vi "Read Old.vi"(5 "channel list":string="BL_SELs", 6 "current limit range (A)":dbl=3.2e-05 format="%#_6p", 7 "aperture time (s)":dbl=0.0005 format="%#_6p", 8 "error in (no error)":errorcluster, 9 "settling time (s)":dbl=0.001 format="%#_6p", 10 "voltage level (V)":dbl=0.2 format="%#_6p", 11 "instrument handle":refnum<k15>="PXI1Slot2 (8)") -> (0 "error out":errorcluster, 1 "currents (A)":dbl[](array[numeric])=[9.855399817894821e-07, -1.469813883694186e-08, -9.562873863260234e-08, -9.678400506461213e-09, -4.0653341648640705e-08, -1.6774881378946392e-08, 2.609795137832926e-09, -3.578297908247983e-08], 2 "resistances (ohm)":dbl[](array[numeric])=[101467.21781741035, -6803582.488189799, -1045710.7500308217, -10332285.787640315, -2459822.3896151385, -5961294.016988207, 38317183.80893152, -2794624.7787111253], 3 "instrument handle out":refnum<k15>="PXI1Slot2 (8)")   [LabVIEW 2018]
uses:
  <instrlib>/niDigital/niDigital.llb/niDigital Selected Function.ctl
  Globals.vi
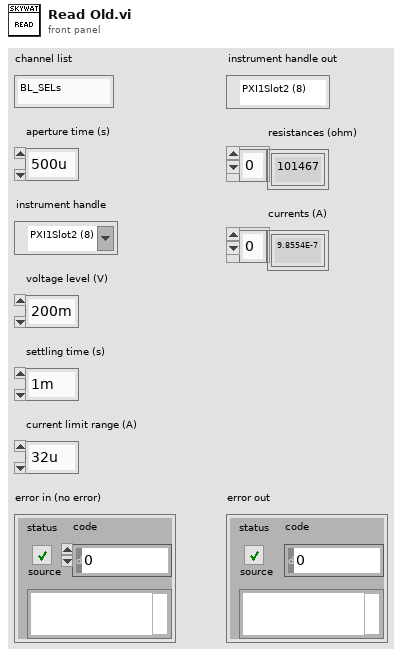
[diagram p1: front panel]
types:
  T1 = typedef "niDigital Selected Function.ctl" = i32
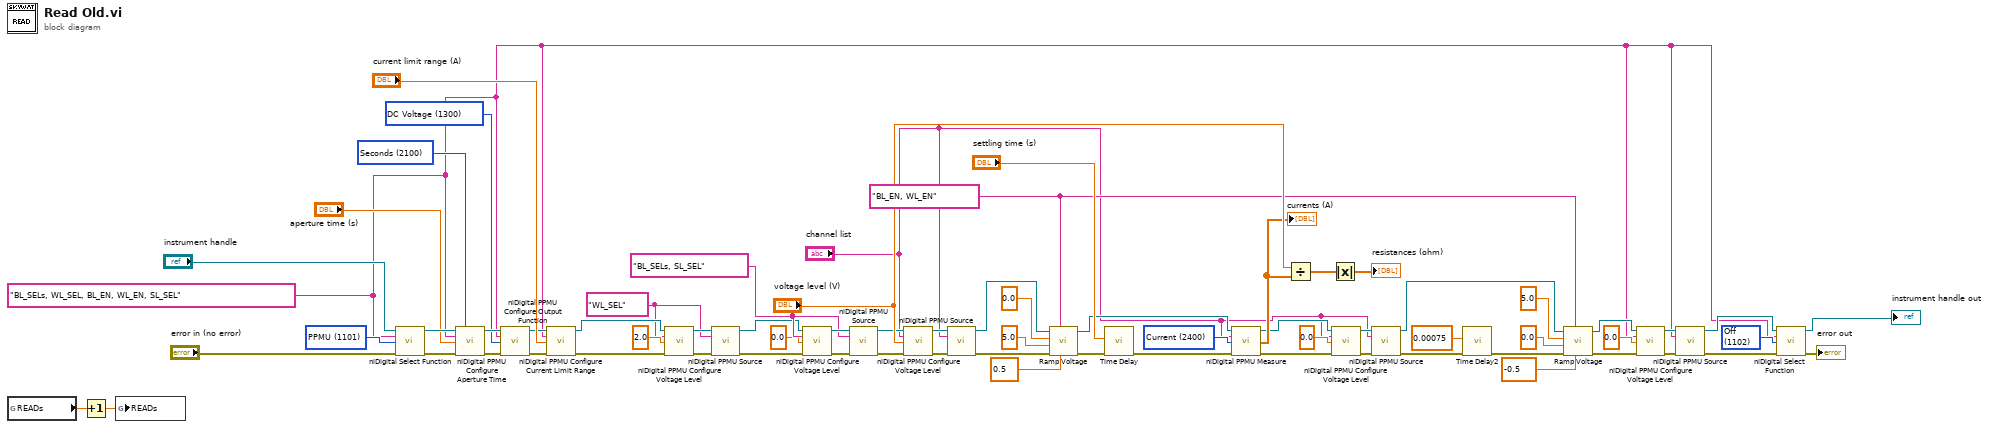
[diagram p0: block diagram]
diagram:
  w14 = "WL_SEL" ("channel list")
  w29 = "BL_EN, WL_EN" ("channel list")
  w49 = "BL_SELs, SL_SEL" ("channel list")
  w4 = "BL_SELs, WL_SEL, BL_EN, WL_EN, SL_SEL" ("channel list")
  w38 = T1 1102 items=["Digital"=1100, "PPMU"=1101, "Off"=1102, "Disconnect"=1103] ("function")
  w58 = u16 2400 items=["Voltage"=2401, "Current"=2400] ("measurement type")
  w68 = T1 1101 items=["Digital"=1100, "PPMU"=1101, "Off"=1102, "Disconnect"=1103] ("function")
  w59 = u16 2100 items=["Seconds"=2100] ("aperture time units")
  w61 = u16 1300 items=["DC Voltage"=1300, "DC Current"=1301] ("output function")
  n1 = global read "Globals.vi" "READs"() -> (w23:dbl)
  n2 = Increment(x=w23) -> (x+1=w22:dbl)
  n3 = global write "Globals.vi" "READs"(w22) -> ()
  n4 = call <instrlib>:"niDigital Select Function.vi"("instrument handle"="instrument handle", "channel list"=w4, "function"=w68, "error in"="error in (no error)") -> ("instrument handle out"=w66:refnum<k15>, "error out"=w67:errorcluster)  [unwired: 10 in]
  n5 = call <instrlib>:"niDigital PPMU Configure Aperture Time.vi"("instrument handle"=w66, "aperture time units"=w59, "channel list"=w4, "aperture time"="aperture time (s)", "error in"=w67) -> ("instrument handle out"=w63:refnum<k15>, "error out"=w64:errorcluster)  [unwired: 9 in]
  n6 = call <instrlib>:"niDigital PPMU Configure Output Function.vi"("instrument handle"=w63, "channel list"=w4, "output function"=w61, "error in"=w64) -> ("instrument handle out"=w60:refnum<k15>, "error out"=w62:errorcluster)  [unwired: 10 in]
  n7 = call <instrlib>:"niDigital PPMU Configure Current Limit Range.vi"("instrument handle"=w60, "channel list"=w4, "current limit range (A)"="current limit range (A)", "error in"=w62) -> ("instrument handle out"=w18:refnum<k15>, "error out"=w17:errorcluster)  [unwired: 10 in]
  n8 = call <instrlib>:"niDigital PPMU Configure Voltage Level.vi"("instrument handle"=w18, "channel list"=w14, "voltage level (V)"=2.0, "error in"=w17) -> ("instrument handle out"=w15:refnum<k15>, "error out"=w16:errorcluster)  [unwired: 10 in]
  n9 = call <instrlib>:"niDigital PPMU Source.vi"("instrument handle"=w15, "channel list"=w14, "error in"=w16) -> ("instrument handle out"=w13:refnum<k15>, "error out"=w12:errorcluster)  [unwired: 11 in]
  n10 = call <instrlib>:"niDigital PPMU Configure Voltage Level.vi"("instrument handle"=w13, "channel list"=w49, "voltage level (V)"=0.0, "error in"=w12) -> ("instrument handle out"=w51:refnum<k15>, "error out"=w52:errorcluster)  [unwired: 10 in]
  n11 = call <instrlib>:"niDigital PPMU Source.vi"("instrument handle"=w51, "channel list"=w49, "error in"=w52) -> ("instrument handle out"=w50:refnum<k15>, "error out"=w48:errorcluster)  [unwired: 11 in]
  n12 = call <instrlib>:"niDigital PPMU Configure Voltage Level.vi"("instrument handle"=w50, "channel list"="channel list", "voltage level (V)"="voltage level (V)", "error in"=w48) -> ("instrument handle out"=w57:refnum<k15>, "error out"=w56:errorcluster)  [unwired: 10 in]
  n13 = call <instrlib>:"niDigital PPMU Source.vi"("instrument handle"=w57, "channel list"="channel list", "error in"=w56) -> ("instrument handle out"=w47:refnum<k15>, "error out"=w46:errorcluster)  [unwired: 11 in]
  n14 = call "Ramp Voltage.vi"("Step"=0.5, "channel list"=w29, "error in (no error)"=w46, "Final Value"=5.0, "Initial Value"=0.0, "instrument handle"=w47) -> ("error out"=w44:errorcluster, "instrument handle out"=w45:refnum<k15>)  [unwired: 4 in]
  n15 = call "Time Delay"("error in (no error)"=w44, "Delay Time (s)"="settling time (s)") -> ("error out"=w70:errorcluster)  [unwired: 9 in]
  n16 = call <instrlib>:"niDigital PPMU Measure.vi"("instrument handle"=w45, "channel list"="channel list", "measurement type"=w58, "error in"=w70) -> ("instrument handle out"=w37:refnum<k15>, "measurements"=w39:dbl[], "error out"=w24:errorcluster)  [unwired: 9 in]
  "currents (A)" <- w39
  n17 = Divide(x="voltage level (V)", y=w39) -> (x/y=w2:dbl[])
  n18 = Absolute Value(x=w2) -> (abs(x)=→"resistances (ohm)":dbl[])
  n19 = call <instrlib>:"niDigital PPMU Configure Voltage Level.vi"("instrument handle"=w37, "channel list"="channel list", "voltage level (V)"=0.0, "error in"=w24) -> ("instrument handle out"=w26:refnum<k15>, "error out"=w25:errorcluster)  [unwired: 10 in]
  n20 = call <instrlib>:"niDigital PPMU Source.vi"("instrument handle"=w26, "channel list"="channel list", "error in"=w25) -> ("instrument handle out"=w30:refnum<k15>, "error out"=w36:errorcluster)  [unwired: 11 in]
  n21 = call "Time Delay2"("error in (no error)"=w36, "Delay Time (s)"=0.00075) -> ("error out"=w31:errorcluster)  [unwired: 9 in]
  n22 = call "Ramp Voltage.vi"("Step"=-0.5, "channel list"=w29, "error in (no error)"=w31, "Final Value"=0.0, "Initial Value"=5.0, "instrument handle"=w30) -> ("error out"=w7:errorcluster, "instrument handle out"=w8:refnum<k15>)  [unwired: 4 in]
  n23 = call <instrlib>:"niDigital PPMU Configure Voltage Level.vi"("instrument handle"=w8, "channel list"=w4, "voltage level (V)"=0.0, "error in"=w7) -> ("instrument handle out"=w10:refnum<k15>, "error out"=w9:errorcluster)  [unwired: 10 in]
  n24 = call <instrlib>:"niDigital PPMU Source.vi"("instrument handle"=w10, "channel list"=w4, "error in"=w9) -> ("instrument handle out"=w6:refnum<k15>, "error out"=w5:errorcluster)  [unwired: 11 in]
  n25 = call <instrlib>:"niDigital Select Function.vi"("instrument handle"=w6, "channel list"=w4, "function"=w38, "error in"=w5) -> ("instrument handle out"=→"instrument handle out":refnum<k15>, "error out"=→"error out":errorcluster)  [unwired: 10 in]
